vi "Spawn.vi"(6 "Start Direction":T1=enum."E", 8 "error in (no error)":errorcluster, 10 "?":T2, 11 "Mother in":refnum<class "Formics.lvclass">) -> (0 "error out":errorcluster, 2 "Replicated Class":refnum<class "Formics.lvclass">, 3 "Mother out":refnum<class "Formics.lvclass">)   [LabVIEW 2014, in "Formics.lvclass"]
uses:
  Formics.lvclass
  Formic Types.ctl
  SquareBattle Arena/Direction Enum.ctl
  Formics.lvclass/Formics.ctl
  Scout/Scout.lvclass
  Coward Options.ctl
  Protector/Protector.lvclass
  SquareBattle Arena/SquareBattle Arena.lvclass
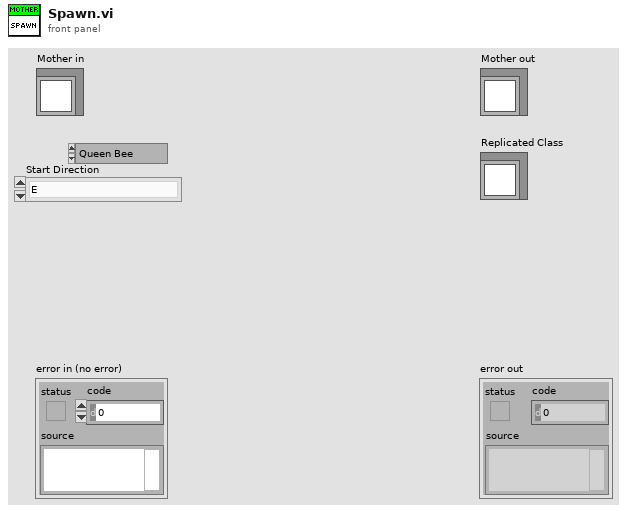
[diagram p1: front panel]
types:
  T1 = typedef "SquareBattle Arena.lvlib/SquareBattle Arena.lvclass/Direction Enum.ctl" = enum16{"NW", "N", "NE", "E", "SE", "S", "SW", "W"}
  T2 = typedef "Formics.lvclass/Formic Types.ctl" = enum16{"Queen Bee", "Protector Bee", "Daughter Bee", "Worker Bee", "Coward"}
  T3 = enum16{"Queen", "Daughter", "Kamikazee", "Coward", "Migrate", "Line Up"}
  T4 = typedef "Formics.lvclass/Coward Options.ctl" = enum16{"Default", "Attack behind and continue", "Attack behind and retreat", "Move Back", "Check if still there"}
  T5 = typedef "Formics.lvclass/SquareStatus DVR.ctl" = refnum<data-value>
  T6 = typedef "Formics.lvclass/Kamikaze DVR.ctl" = refnum<data-value>
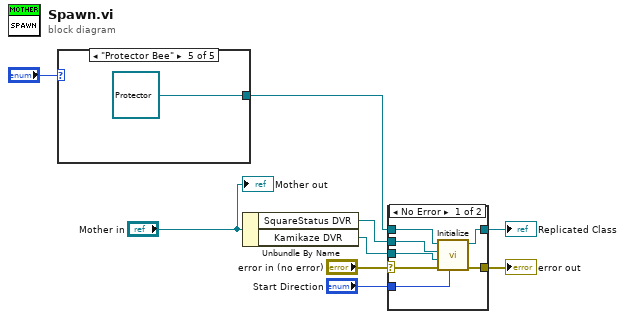
[diagram p0: block diagram]
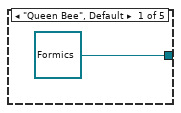
[diagram p2: hidden frame]
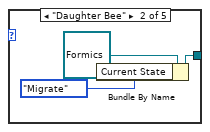
[diagram p3: hidden frame]
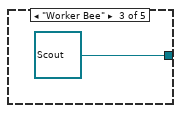
[diagram p4: hidden frame]
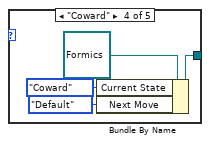
[diagram p5: hidden frame]
diagram:
  n1 = case shown="\"Protector Bee\"" "?" {
    tunnel: [refnum<class "Formics.lvclass"> refnum ("Mother.lvclass") w12 refnum<class "Scout.lvclass"> refnum ("Scout.lvclass") w17 refnum<class "Protector.lvclass"> refnum ("Protector.lvclass")] -> w6
    frame "Queen Bee", Default {
    }
    frame "Daughter Bee" {
      n2 = Bundle By Name(cluster=refnum<class "Formics.lvclass"> refnum ("Mother.lvclass"), "Current State"=T3."Migrate") -> (w12:refnum<class "Formics.lvclass">)
    }
    frame "Worker Bee" {
    }
    frame "Coward" {
      n3 = Bundle By Name(cluster=refnum<class "Formics.lvclass"> refnum ("Formics.lvclass"), "Current State"=T3."Coward", "Next Move"=Coward_Options."Default") -> (w17:refnum<class "Formics.lvclass">)
    }
    frame "Protector Bee" {
    }
  }
  n4 = Unbundle By Name("Mother in") -> ("SquareStatus DVR"=w3:T5, "Kamikaze DVR"=w2:T6)
  n5 = case shown="No Error" "error in (no error)" {
    selector: "error in (no error)" -> [w26 w28]
    tunnel: [w25 w28] -> w8
    tunnel: [w23 w27] -> w5
    tunnel: w6 -> [w24 w27]
    tunnel: w3 -> [w22 _]
    tunnel: w2 -> [w21 _]
    tunnel: "Start Direction" -> [w20 _]
    frame No Error {
      n6 = call-dynamic "Initialize.vi"("Start Direction"=w20, "error in (no error)"=w26, "Kamikaze DVR"=w21, "SquareStatus DVR"=w22, "Mother in"=w24) -> ("error out"=w25:errorcluster, "Mother out"=w23:refnum<class "Formics.lvclass">)  [unwired: 5 in]
    }
    frame Error {
    }
  }
  "error out" <- w8
  "Replicated Class" <- w5
  "Mother out" <- "Mother in"
